vi "Update State Data.vi"(8 "error in (no error)":errorcluster, 9 "Data":variant, 10 "Argument":string, 11 "State Data":T1) -> (0 "error out":errorcluster, 3 "State Data out":T1)   [LabVIEW 2023, in "VI Properties Editor.lvlib"]
uses:
  VI Properties Editor.lvlib
  <vilib>/Utility/error.llb/Error Cluster From Error Code.vi
  <vilib>/ErrorRing/Error Ring.xnode
  3573416a-ab14-40fa-8eb1-e5c23e8662a1.vi
  6c3ab29c-e086-46da-822f-1f7a3bdde8cc.vi
  CTLs/Filter Column.ctl
  CTLs/Filter Type.ctl
  <vilib>/picture/picture.llb/imagedata.ctl
  CTLs/VI Properties.ctl
  CTLs/Control Properties.ctl
  CTLs/VI Data.ctl
  CTLs/Main Front Panel Controls.ctl
  CTLs/Config.ctl
  <vilib>/Utility/miscctls.llb/LVSelectionTypeDef.ctl
  CTLs/Filter.ctl
  CTLs/Main References.ctl
  CTLs/Main State Data.ctl
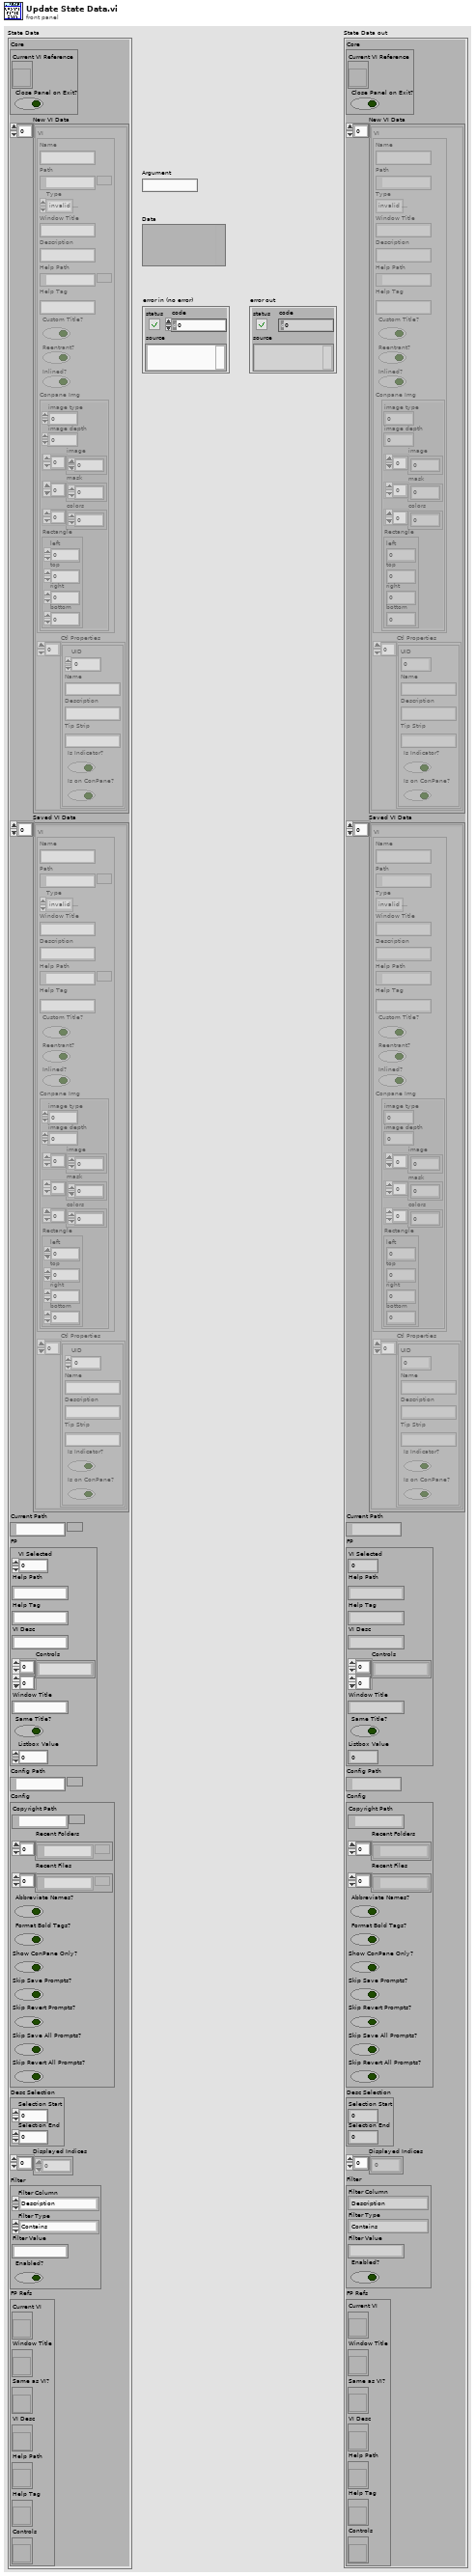
[diagram p1: front panel]
types:
  T1 = typedef "VI Properties Editor.lvlib/Main State Data.ctl" = cluster{"Core":cluster{"Current VI Reference":refnum<vi>, "Close Panel on Exit?":bool}, "New VI Data":T2[], "Saved VI Data":T2[], "Current Path":path, "FP":T6, "Config Path":path, "Config":T7, "Desc Selection":T8, "Displayed Indices":i32[], "Filter":T9, "FP Refs":T12}
  T2 = typedef "VI Properties Editor.lvlib/VI Data.ctl" = cluster{"VI":T3, "Ctl Properties":T5[]}
  T3 = typedef "VI Properties Editor.lvlib/VI Properties.ctl" = cluster{"Name":string, "Path":path, "Type":enum32{"invalid VI type", "Standard VI", "Control VI", "Global VI", "Polymorphic VI", "Configuration VI", "SubSystem", "Facade VI", "Method VI", "Statechart Diagram VI"}, "Window Title":string, "Description":string, "Help Path":path, "Help Tag":string, "Custom Title?":bool, "Reentrant?":bool, "Inlined?":bool, "Conpane Img":T4}
  T4 = typedef "imagedata.ctl" = cluster{"image type":i32, "image depth":i32, "image":u8[], "mask":u8[], "colors":u32[], "Rectangle":cluster{"left":i16, "top":i16, "right":i16, "bottom":i16}}
  T5 = typedef "VI Properties Editor.lvlib/Control Properties.ctl" = cluster{"UID":i32, "Name":string, "Description":string, "Tip Strip":string, "Is Indicator?":bool, "Is on ConPane?":bool}
  T6 = typedef "VI Properties Editor.lvlib/Main Front Panel Controls.ctl" = cluster{"VI Selected":i32, "Help Path":string, "Help Tag":string, "VI Desc":string, "Controls":string[][], "Window Title":string, "Same Title?":bool, "Listbox Value":i32}
  T7 = typedef "VI Properties Editor.lvlib/Config.ctl" = cluster{"Copyright Path":path, "Recent Folders":path[], "Recent Files":path[], "Abbreviate Names?":bool, "Format Bold Tags?":bool, "Show ConPane Only?":bool, "Skip Save Prompts?":bool, "Skip Revert Prompts?":bool, "Skip Save All Prompts?":bool, "Skip Revert All Prompts?":bool}
  T8 = typedef "LVSelectionTypeDef.ctl" = cluster{"Selection Start":u32, "Selection End":u32}
  T9 = typedef "VI Properties Editor.lvlib/Filter.ctl" = cluster{"Filter Column":T10, "Filter Type":T11, "Filter Value":string, "Enabled?":bool}
  T10 = typedef "VI Properties Editor.lvlib/Filter Column.ctl" = enum16{"Description"}
  T11 = typedef "VI Properties Editor.lvlib/Filter Type.ctl" = enum16{"Contains", "Equals", "Starts with", "Ends with", "Does not contain", "Does not equal", "Is empty", "Is not empty"}
  T12 = typedef "VI Properties Editor.lvlib/Main References.ctl" = cluster{"Current VI":refnum<vi>, "Window Title":refnum<vi>, "Same as VI?":refnum<vi>, "VI Desc":refnum<vi>, "Help Path":refnum<vi>, "Help Tag":refnum<vi>, "Controls":refnum<vi>}
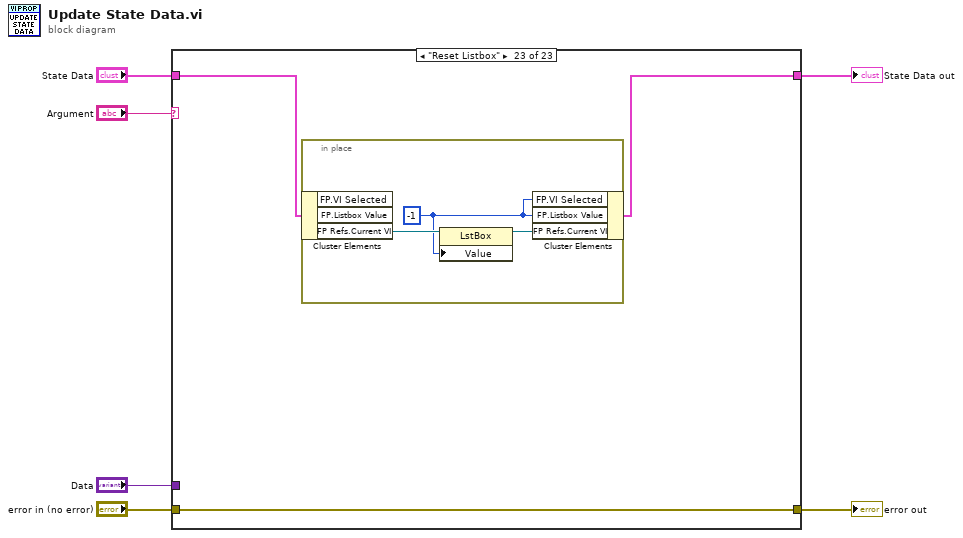
[diagram p0: block diagram]
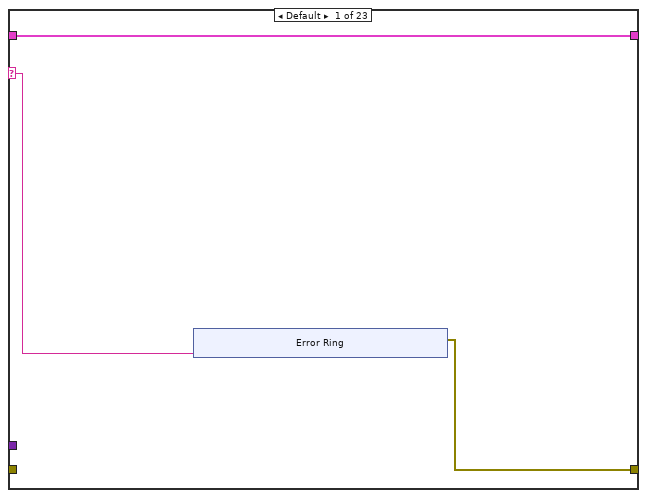
[diagram p2: hidden frame]
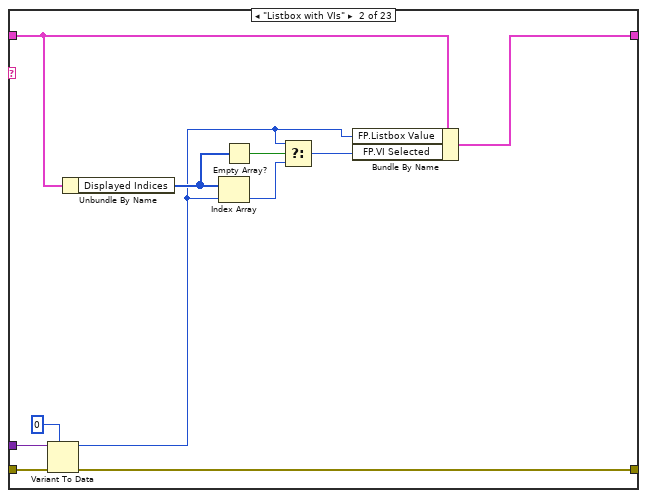
[diagram p3: hidden frame]
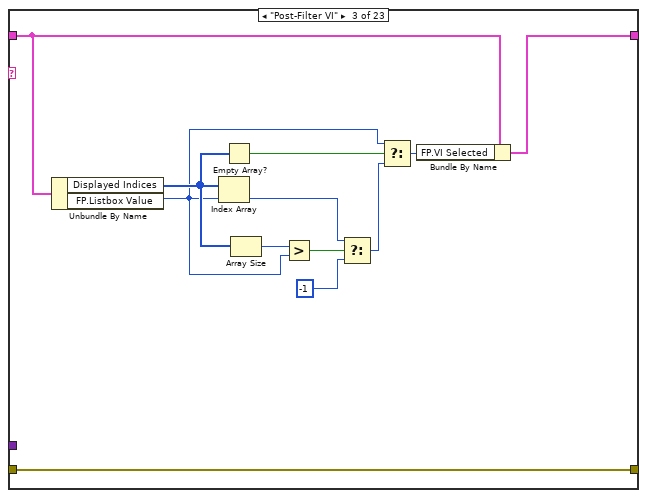
[diagram p4: hidden frame]
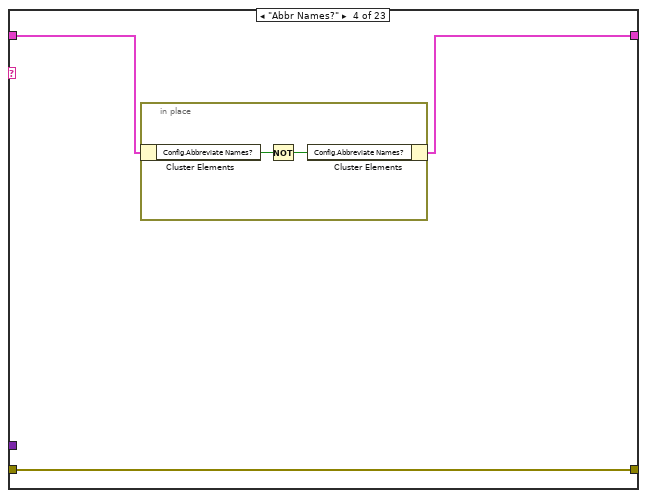
[diagram p5: hidden frame]
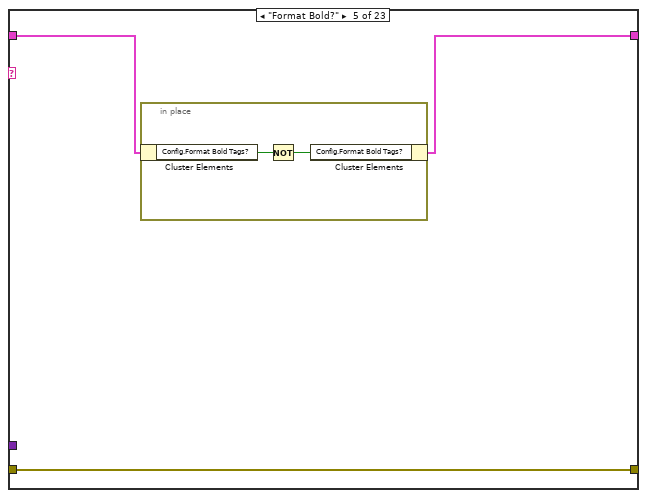
[diagram p6: hidden frame]
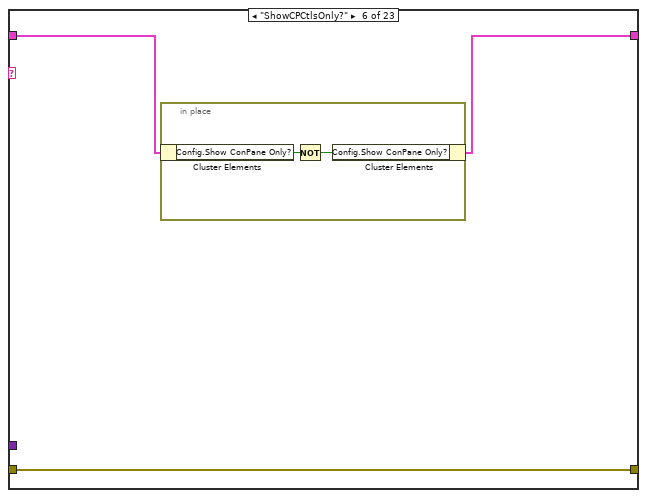
[diagram p7: hidden frame]
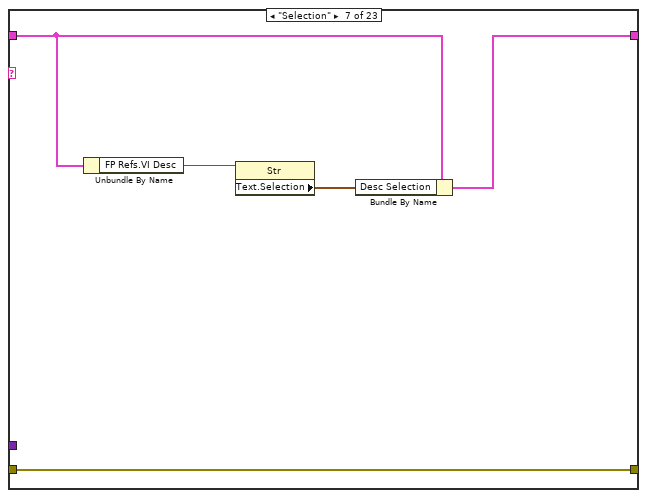
[diagram p8: hidden frame]
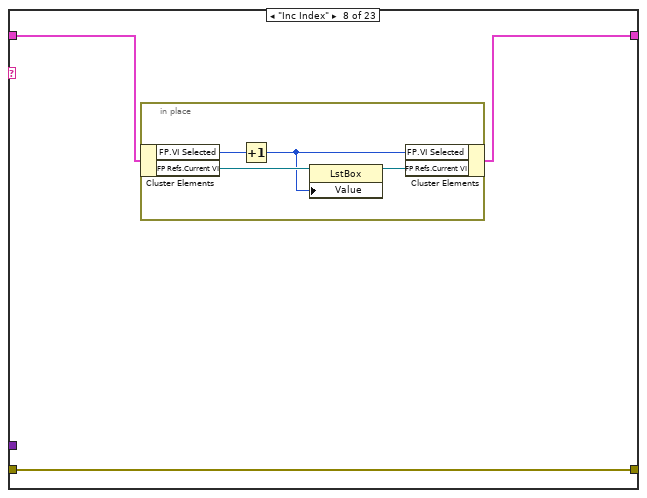
[diagram p9: hidden frame]
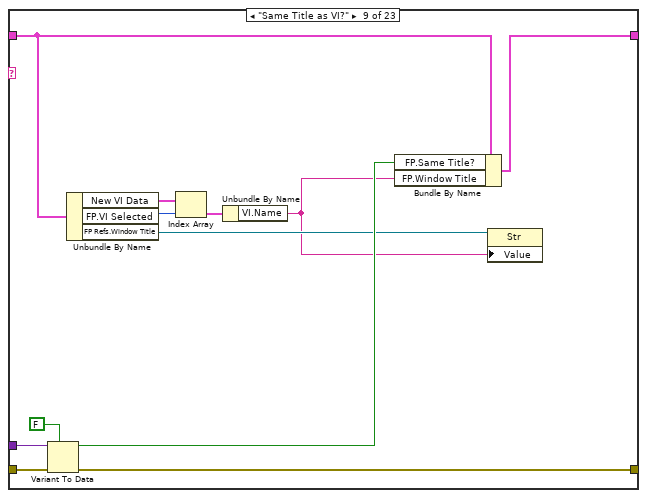
[diagram p10: hidden frame]
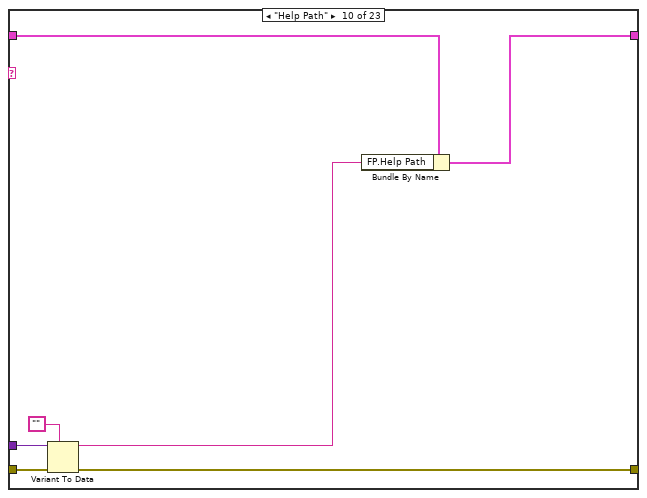
[diagram p11: hidden frame]
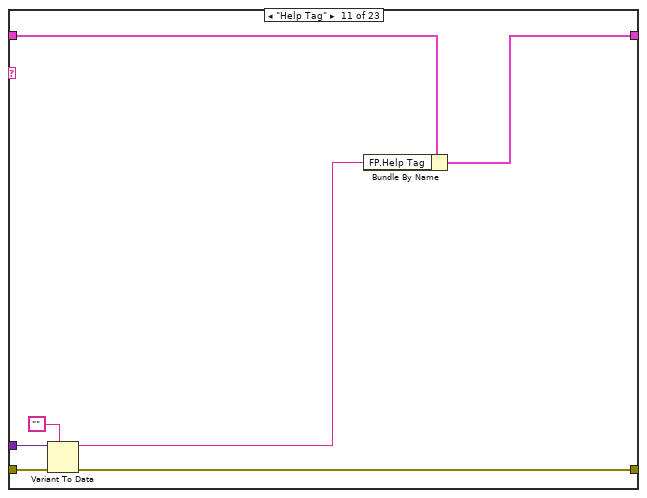
[diagram p12: hidden frame]
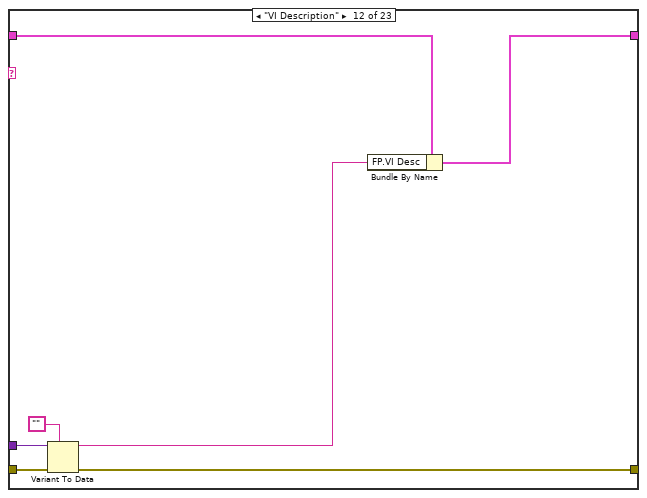
[diagram p13: hidden frame]
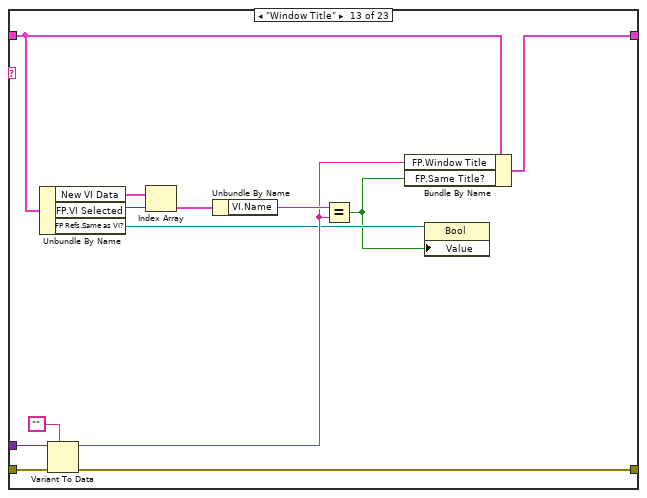
[diagram p14: hidden frame]
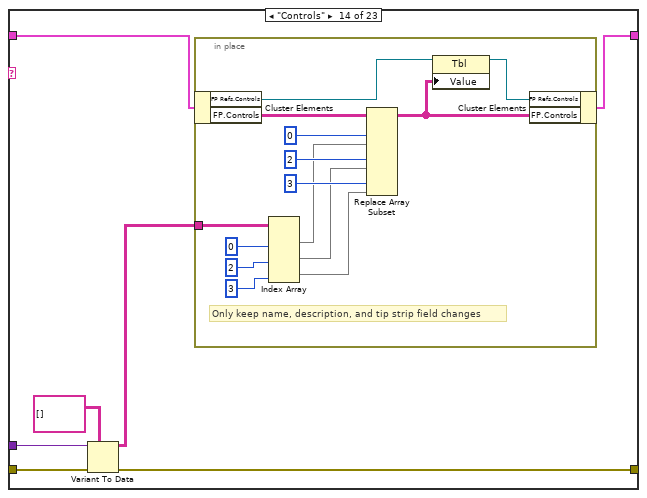
[diagram p15: hidden frame]
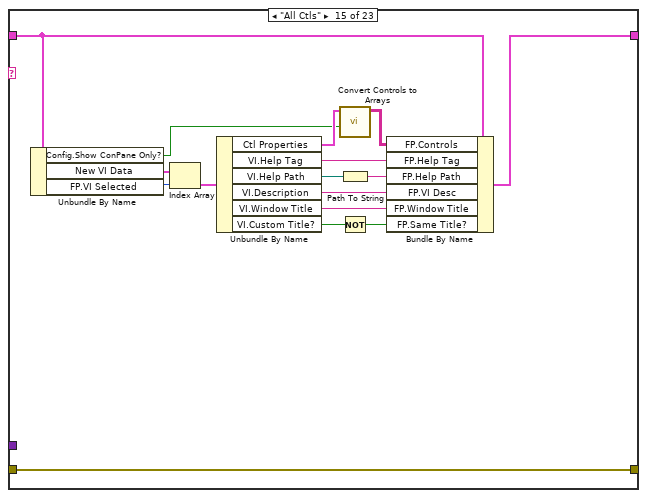
[diagram p16: hidden frame]
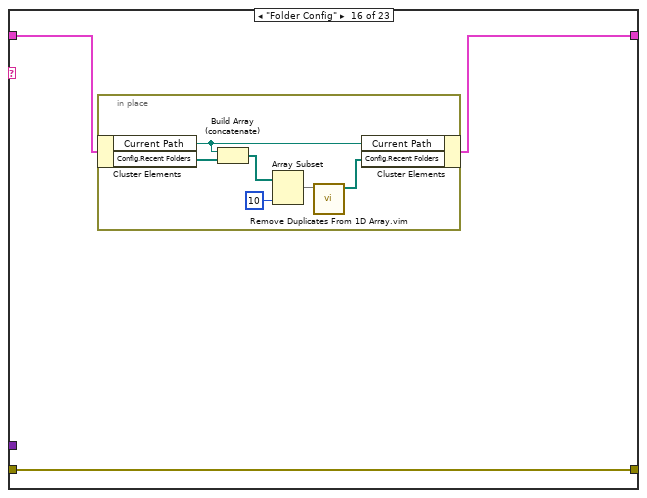
[diagram p17: hidden frame]
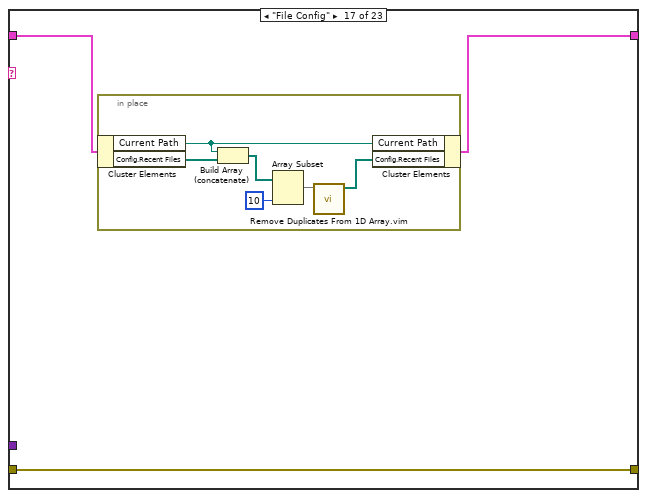
[diagram p18: hidden frame]
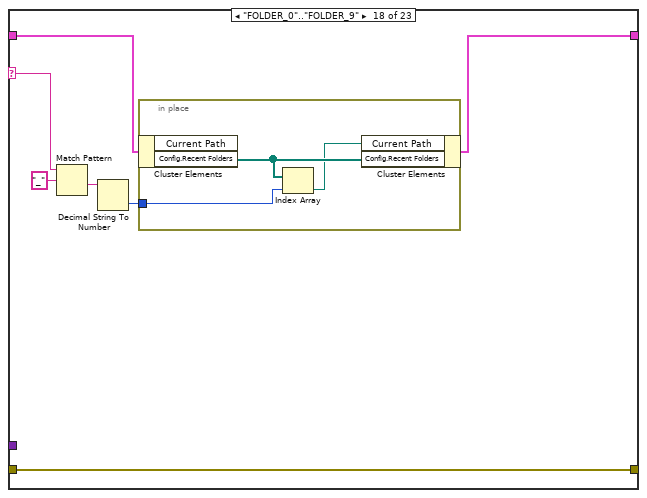
[diagram p19: hidden frame]
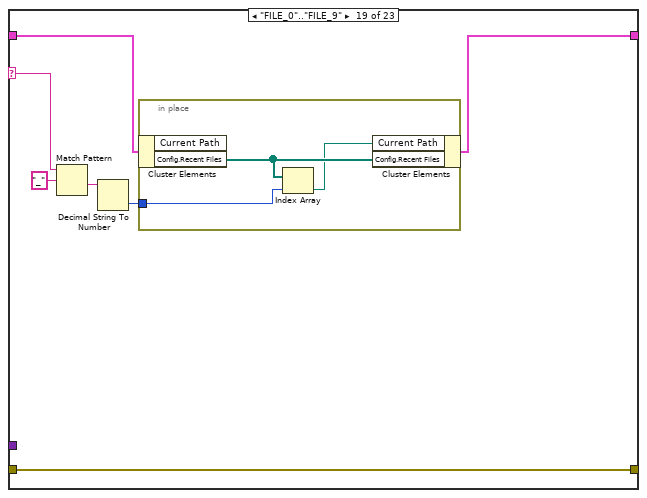
[diagram p20: hidden frame]
diagram:
  n1 = case shown="\"Reset Listbox\"" "Argument" {
    selector: "Argument" -> [w8 _ _ _ _ _ _ _ _ _ _ _ _ _ _ _ _ w172 w182 _ _ _ _]
    tunnel: "error in (no error)" -> [_ w27 w36 w42 w47 w52 w59 w62 w78 w85 w92 w99 w112 w119 w147 w152 w161 w174 w184 w190 w196 w203 w207]
    tunnel: "State Data" -> [w9 w22 w38 w41 w46 w51 w56 w61 w69 w82 w89 w96 w105 w115 w148 w150 w159 w168 w178 w188 w194 w201 w205]
    tunnel: "Data" -> [_ w26 _ _ _ _ _ _ w77 w84 w91 w98 w111 w118 _ _ _ _ _ _ _ _ _]
    tunnel: [w7 w24 w36 w42 w47 w52 w59 w62 w74 w80 w87 w94 w109 w117 w147 w152 w161 w174 w184 w190 w196 w203 w207] -> w1
    tunnel: [w9 w23 w39 w40 w45 w50 w57 w60 w73 w79 w86 w93 w108 w113 w149 w151 w160 w173 w183 w189 w195 w202 w206] -> w5
    frame Default {
      n2 = xnode "Error Ring"("parameter 0"=w8) -> ("error out"=w7:errorcluster)
    }
    frame "Listbox with VIs" {
      n3 = Variant To Data(error in=w27, type=0, Variant=w26) -> (data=w17:i32, error out=w24:errorcluster)
      n4 = Unbundle By Name(w22) -> ("Displayed Indices"=w21:i32[])
      n5 = Index Array(array=w21, index=w17) -> (element=w19:i32)
      n6 = Empty Array?(array=w21) -> (empty?=w20:bool)
      n7 = Select(t=w17, s=w20, f=w19) -> (s? t:f=w18:i32)
      n8 = Bundle By Name(cluster=w22, "FP.Listbox Value"=w17, "FP.VI Selected"=w18) -> (w23:T1)
    }
    frame "Post-Filter VI" {
      n9 = Unbundle By Name(w38) -> ("Displayed Indices"=w35:i32[], "FP.Listbox Value"=w33:i32)
      n10 = Index Array(array=w35, index=w33) -> (element=w30:i32)
      n11 = Empty Array?(array=w35) -> (empty?=w37:bool)
      n12 = Array Size(array=w35) -> (size(s)=w34:i32)
      n13 = Greater?(x=w34, y=w33) -> (0:w32:bool)
      n14 = Select(t=w30, s=w32, f=-1) -> (s? t:f=w28:i32)
      n15 = Select(t=w33, s=w37, f=w28) -> (s? t:f=w29:i32)
      n16 = Bundle By Name(cluster=w38, "FP.VI Selected"=w29) -> (w39:T1)
    }
    frame "Abbr Names?" {
      n17 = in-place {
        n18 = in-place-cluster #1(w41) -> ("Config.Abbreviate Names?"=w44:bool)
        n19 = Not(x=w44) -> (.not. x?=w43:bool)
        n20 = in-place-cluster #1("Config.Abbreviate Names?"=w43) -> (w40:T1)
      }
    }
    frame "Format Bold?" {
      n21 = in-place {
        n22 = in-place-cluster #2(w46) -> ("Config.Format Bold Tags?"=w49:bool)
        n23 = Not(x=w49) -> (.not. x?=w48:bool)
        n24 = in-place-cluster #2("Config.Format Bold Tags?"=w48) -> (w45:T1)
      }
    }
    frame "ShowCPCtlsOnly?" {
      n25 = in-place {
        n26 = in-place-cluster #3(w51) -> ("Config.Show ConPane Only?"=w54:bool)
        n27 = Not(x=w54) -> (.not. x?=w53:bool)
        n28 = in-place-cluster #3("Config.Show ConPane Only?"=w53) -> (w50:T1)
      }
    }
    frame "Selection" {
      n29 = Unbundle By Name(w56) -> ("FP Refs.VI Desc"=w55:refnum<vi>)
      n30 = property on="Property Node" class="Str"(reference=w55) -> ("Text.Selection"=w58:T8)  [unwired: 1 in, 2 out]
      n31 = Bundle By Name(cluster=w56, "Desc Selection"=w58) -> (w57:T1)
    }
    frame "Inc Index" {
      n32 = in-place {
        n33 = in-place-cluster #4(w61) -> ("FP.VI Selected"=w66:i32, "FP Refs.Current VI"=w65:refnum<vi>)
        n34 = Increment(x=w66) -> (x+1=w63:i32)
        n35 = property class="LstBox"(reference=w65, "Value"=w63) -> (reference out=w64:refnum<vi>)  [unwired: 1 in, 1 out]
        n36 = in-place-cluster #4("FP.VI Selected"=w63, "FP Refs.Current VI"=w64) -> (w60:T1)
      }
    }
    frame "Same Title as VI?" {
      n37 = Variant To Data(error in=w78, type=FALSE, Variant=w77) -> (data=w75:bool, error out=w74:errorcluster)
      n38 = Unbundle By Name(w69) -> ("New VI Data"=w72:T2[], "FP.VI Selected"=w71:i32, "FP Refs.Window Title"=w68:refnum<vi>)
      n39 = Index Array(array=w72, index=w71) -> (element=w70:T2)
      n40 = Unbundle By Name(w70) -> ("VI.Name"=w67:string)
      n41 = Bundle By Name(cluster=w69, "FP.Same Title?"=w75, "FP.Window Title"=w67) -> (w73:T1)
      n42 = property class="Str"(reference=w68, "Value"=w67) -> ()  [unwired: 1 in, 2 out]
    }
    frame "Help Path" {
      n43 = Variant To Data(error in=w85, type="", Variant=w84) -> (data=w81:string, error out=w80:errorcluster)
      n44 = Bundle By Name(cluster=w82, "FP.Help Path"=w81) -> (w79:T1)
    }
    frame "Help Tag" {
      n45 = Variant To Data(error in=w92, type="", Variant=w91) -> (data=w88:string, error out=w87:errorcluster)
      n46 = Bundle By Name(cluster=w89, "FP.Help Tag"=w88) -> (w86:T1)
    }
    frame "VI Description" {
      n47 = Variant To Data(error in=w99, type="", Variant=w98) -> (data=w95:string, error out=w94:errorcluster)
      n48 = Bundle By Name(cluster=w96, "FP.VI Desc"=w95) -> (w93:T1)
    }
    frame "Window Title" {
      n49 = Unbundle By Name(w105) -> ("New VI Data"=w107:T2[], "FP.VI Selected"=w106:i32, "FP Refs.Same as VI?"=w101:refnum<vi>)
      n50 = Variant To Data(error in=w112, type="", Variant=w111) -> (data=w102:string, error out=w109:errorcluster)
      n51 = Index Array(array=w107, index=w106) -> (element=w104:T2)
      n52 = Unbundle By Name(w104) -> ("VI.Name"=w103:string)
      n53 = Equal?(x=w103, y=w102) -> (x = y?=w100:bool)
      n54 = Bundle By Name(cluster=w105, "FP.Window Title"=w102, "FP.Same Title?"=w100) -> (w108:T1)
      n55 = property class="Bool"(reference=w101, "Value"=w100) -> ()  [unwired: 1 in, 2 out]
    }
    frame "Controls" {
      n56 = Variant To Data(error in=w119, type=string[][] [], Variant=w118) -> (data=w114:string[][], error out=w117:errorcluster)
      n57 = in-place {
        in-place-border: w114 -> [w133]
        # "Only keep name, description, and tip strip field changes"
        n58 = in-place-cluster #5(w115) -> ("FP Refs.Controls"=w122:refnum<vi>, "FP.Controls"=w132:string[][])
        n59 = Index Array(array=w133, index (col) #1=0 ("disabled index (col)"), index (col) #2=2 ("index (row)"), index (col) #3=3 ("index (row)")) -> (element #1=w125:string[], element #2=w124:string[], element #3=w123:string[])  [unwired: 3 in]
        n60 = Replace Array Subset(array=w132, new element #1=w125, index (col) #1=0 ("index (row)"), new element #2=w124, index (col) #2=2 ("index (row)"), new element #3=w123, index (col) #3=3 ("index (row)")) -> (w120:string[][])  [unwired: 3 in]
        n61 = property class="Tbl"(reference=w122, "Value"=w120) -> (reference out=w121:refnum<vi>)  [unwired: 1 in, 1 out]
        n62 = in-place-cluster #5("FP Refs.Controls"=w121, "FP.Controls"=w120) -> (w113:T1)
      }
    }
    frame "All Ctls" {
      n63 = Unbundle By Name(w148) -> ("Config.Show ConPane Only?"=w134:bool, "New VI Data"=w146:T2[], "FP.VI Selected"=w145:i32)
      n64 = Index Array(array=w146, index=w145) -> (element=w144:T2)
      n65 = Unbundle By Name(w144) -> ("Ctl Properties"=w135:T5[], "VI.Help Tag"=w139:string, "VI.Help Path"=w141:path, "VI.Description"=w143:string, "VI.Window Title"=w138:string, "VI.Custom Title?"=w137:bool)
      n66 = call "Convert Controls to Arrays.vi"("ConPane Only?"=w134, "Ctl Properties"=w135) -> ("Control Array"=w142:string[][])  [unwired: 9 in]
      n67 = Path To String(path=w141) -> (string=w140:string)
      n68 = Not(x=w137) -> (.not. x?=w136:bool)
      n69 = Bundle By Name(cluster=w148, "FP.Controls"=w142, "FP.Help Tag"=w139, "FP.Help Path"=w140, "FP.VI Desc"=w143, "FP.Window Title"=w138, "FP.Same Title?"=w136) -> (w149:T1)
    }
    frame "Folder Config" {
      n70 = in-place {
        n71 = in-place-cluster #6(w150) -> ("Current Path"=w155:path, "Config.Recent Folders"=w158:path[])
        n72 = Build Array (concatenate)(w155, w158) -> (w157:path[])
        n73 = Array Subset(array=w157, length=10) -> (w154:path[])  [unwired: 1 in]
        n74 = call "Remove Duplicates From 1D Array.vim"("array"=w154) -> ("array with duplicates removed"=w153:path[])  [unwired: 10 in]
        n75 = in-place-cluster #6("Current Path"=w155, "Config.Recent Folders"=w153) -> (w151:T1)
      }
    }
    frame "File Config" {
      n76 = in-place {
        n77 = in-place-cluster #7(w159) -> ("Current Path"=w164:path, "Config.Recent Files"=w167:path[])
        n78 = Build Array (concatenate)(w164, w167) -> (w166:path[])
        n79 = Array Subset(array=w166, length=10) -> (w163:path[])  [unwired: 1 in]
        n80 = call "Remove Duplicates From 1D Array.vim"("array"=w163) -> ("array with duplicates removed"=w162:path[])  [unwired: 10 in]
        n81 = in-place-cluster #7("Current Path"=w164, "Config.Recent Files"=w162) -> (w160:T1)
      }
    }
    frame "FOLDER_0".."FOLDER_9" {
      n82 = Match Pattern(string=w172, regular expression="_") -> (after substring=w170:string)  [unwired: 1 in, 3 out]
      n83 = Decimal String To Number(string=w170) -> (number=w169:i32)  [unwired: 2 in, 1 out]
      n84 = in-place {
        in-place-border: w169 -> [w176]
        n85 = in-place-cluster #8(w168) -> ("Config.Recent Folders"=w177:path[])  [unwired: 1 out]
        n86 = Index Array(array=w177, index=w176) -> (element=w175:path)
        n87 = in-place-cluster #8("Current Path"=w175, "Config.Recent Folders"=w177) -> (w173:T1)
      }
    }
    frame "FILE_0".."FILE_9" {
      n88 = Match Pattern(string=w182, regular expression="_") -> (after substring=w180:string)  [unwired: 1 in, 3 out]
      n89 = Decimal String To Number(string=w180) -> (number=w179:i32)  [unwired: 2 in, 1 out]
      n90 = in-place {
        in-place-border: w179 -> [w186]
        n91 = in-place-cluster #9(w178) -> ("Config.Recent Files"=w187:path[])  [unwired: 1 out]
        n92 = Index Array(array=w187, index=w186) -> (element=w185:path)
        n93 = in-place-cluster #9("Current Path"=w185, "Config.Recent Files"=w187) -> (w183:T1)
      }
    }
    frame "Filter" {
      n94 = in-place {
        n95 = in-place-cluster #10(w188) -> ()  [unwired: 3 out]
        n96 = in-place-cluster #10("Filter.Filter Column"=Filter_Column."Description", "Filter.Filter Type"=Filter_Type."Is empty", "Filter.Enabled?"=TRUE) -> (w189:T1)
      }
    }
    frame "Filter 2" {
      n97 = in-place {
        n98 = in-place-cluster #11(w194) -> ()  [unwired: 4 out]
        n99 = in-place-cluster #11("Filter.Filter Value"="<[Bb]>.+</[Bb]>", "Filter.Filter Column"=Filter_Column."Description", "Filter.Filter Type"=Filter_Type."Does not contain", "Filter.Enabled?"=TRUE) -> (w195:T1)
      }
    }
    frame "Clear Filter" {
      n100 = in-place {
        n101 = in-place-cluster #12(w201) -> ()  [unwired: 1 out]
        n102 = in-place-cluster #12("Filter.Enabled?"=FALSE) -> (w202:T1)
      }
    }
    frame "Reset Listbox" {
      n103 = in-place {
        w208 = -1 ("FP.Listbox Value")
        n104 = in-place-cluster #13(w205) -> ("FP Refs.Current VI"=w210:refnum<vi>)  [unwired: 2 out]
        n105 = property class="LstBox"(reference=w210, "Value"=w208) -> (reference out=w209:refnum<vi>)  [unwired: 1 in, 1 out]
        n106 = in-place-cluster #13("FP.VI Selected"=w208, "FP.Listbox Value"=w208, "FP Refs.Current VI"=w209) -> (w206:T1)
      }
    }
  }
  "State Data out" <- w5
  "error out" <- w1
